vi "Set UI Control Value.vi"(8 "error in (no error)":errorcluster, 10 "VI Ref":refnum<vi>, 11 "I32 Parameter in":refnum<class "I32 Parameter.lvclass">) -> (0 "error out":errorcluster, 3 "I32 Parameter out":refnum<class "I32 Parameter.lvclass">)   [LabVIEW 2016, in "CD Parameter Manager API.lvlib" / "I32 Parameter.lvclass"]
uses:
  I32 Parameter.lvclass
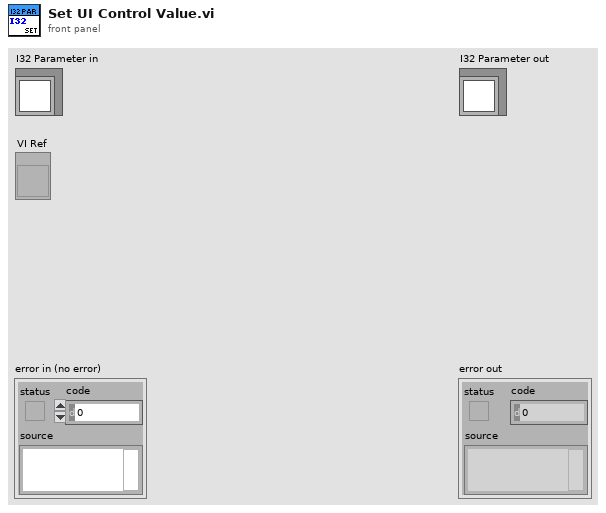
[diagram p1: front panel]
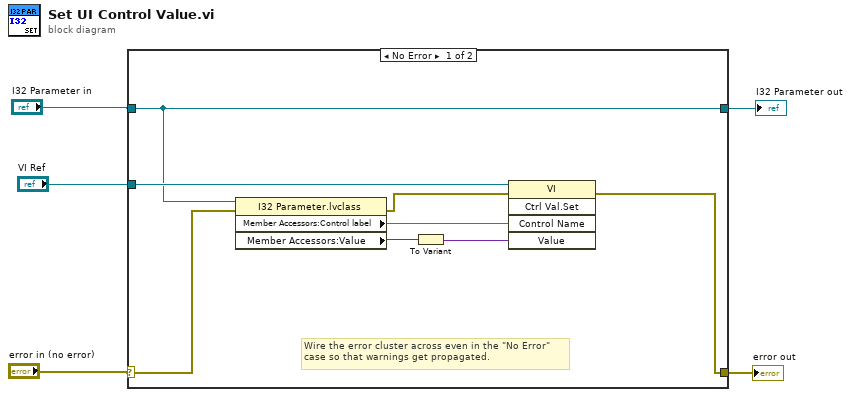
[diagram p0: block diagram]
diagram:
  n1 = case shown="No Error" "error in (no error)" {
    selector: "error in (no error)" -> [w7 w15]
    tunnel: [w11 w15] -> w3
    tunnel: [w10 w14] -> w2
    tunnel: "I32 Parameter in" -> [w10 w14]
    tunnel: "VI Ref" -> [w13 _]
    frame No Error {
      # "Wire the error cluster across even in the \"No Error\"\ncase so that warnings get propagated."
      n2 = property class="I32 Parameter.lvclass"(reference=w10, error in=w7) -> (error out=w6:errorcluster, "Member Accessors:Control label"=w9:string, "Member Accessors:Value"=w8:i32)  [unwired: 1 out]
      n3 = To Variant(anything=w8) -> (Variant=w12:variant)
      n4 = invoke class="VI" method="Ctrl Val.Set"(reference=w13, error in=w6, "Control Name"=w9, "Value"=w12) -> (error out=w11:errorcluster)  [unwired: 1 in, 4 out]
    }
    frame Error {
    }
  }
  "error out" <- w3
  "I32 Parameter out" <- w2
